vi "Burst_test.vi"() -> ()   [LabVIEW 2013, in "VI-Test.lvlib"]
uses:
  Burst.lvclass
  lib/VI-Test.lvlib
panel:
  out "wait":i32[](array[numeric])=[0, 30000, 0, 0]
  out "timeout":u32[](array[numeric])
  out "error out":errorcluster
  out "parameters":string[][](table)
  out "Commandlist":string
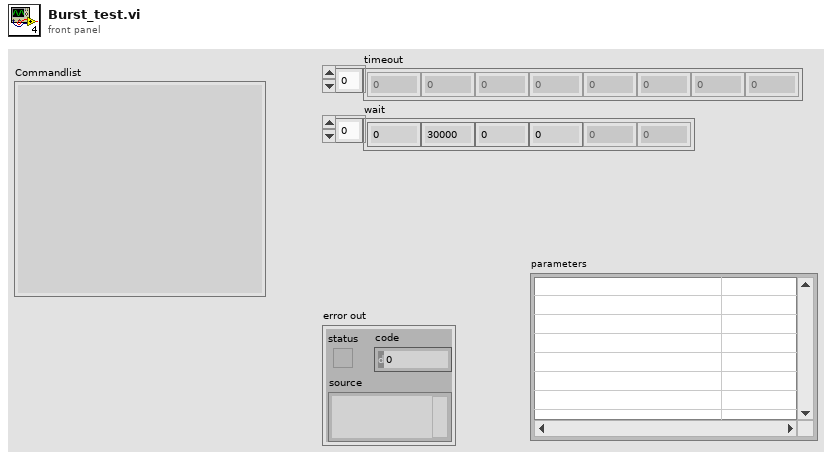
[diagram p1: front panel]
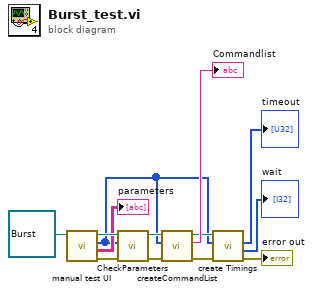
[diagram p0: block diagram]
diagram:
  n1 = call-dynamic "manual test UI.vi"("Burst Eingang"=refnum<class "Burst.lvclass"> refnum) -> ("error out"=w12:errorcluster, "parameters"=→"parameters":string[][], "Parameters"=w4:u32[], "Burst Ausgang"=w13:refnum<class "Burst.lvclass">)  [unwired: 6 in, 1 out]
  n2 = call-dynamic "CheckParameters.vi"("error in (no error)"=w12, "Parameters"=w4, "Burst in"=w13) -> ("error out"=w11:errorcluster, "Burst out"=w8:refnum<class "Burst.lvclass">)  [unwired: 7 in]
  n3 = call-dynamic "createCommandList.vi"("error in (no error)"=w11, "Parameters"=w4, "Burst in"=w8) -> ("error out"=w5:errorcluster, "Commandlist"=→"Commandlist":string, "Burst out"=w6:refnum<class "Burst.lvclass">)  [unwired: 6 in]
  n4 = call-dynamic "create Timings.vi"("error in (no error)"=w5, "Parameters"=w4, "Burst in"=w6) -> ("error out"=→"error out":errorcluster, "wait"=→"wait":i32[], "timeout"=→"timeout":u32[])  [unwired: 5 in, 1 out]
